vi "InitCA.vi"(11 "N-Back":u8) -> (3 "CA":T1(array[cluster]))   [LabVIEW 2020]
uses:
  Global Variables/Global N-Back Setting.vi
  Global Variables/Global Number of Indices.vi
panel:
  in  "New square":T2
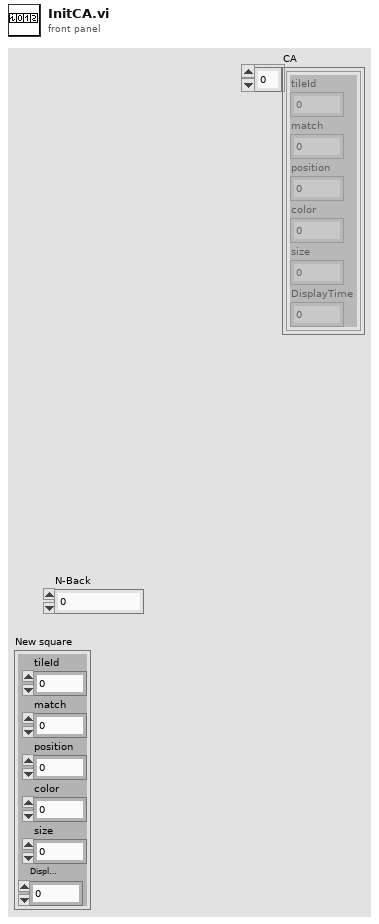
[diagram p1: front panel]
types:
  T1 = cluster{"tileId":i32, "match":i32, "position":i32, "color":u32, "size":i32, "DisplayTime":i32}[]
  T2 = cluster{"tileId":i32, "match":i32, "position":i32, "color":u32, "size":i32, "DisplayTime":i32}
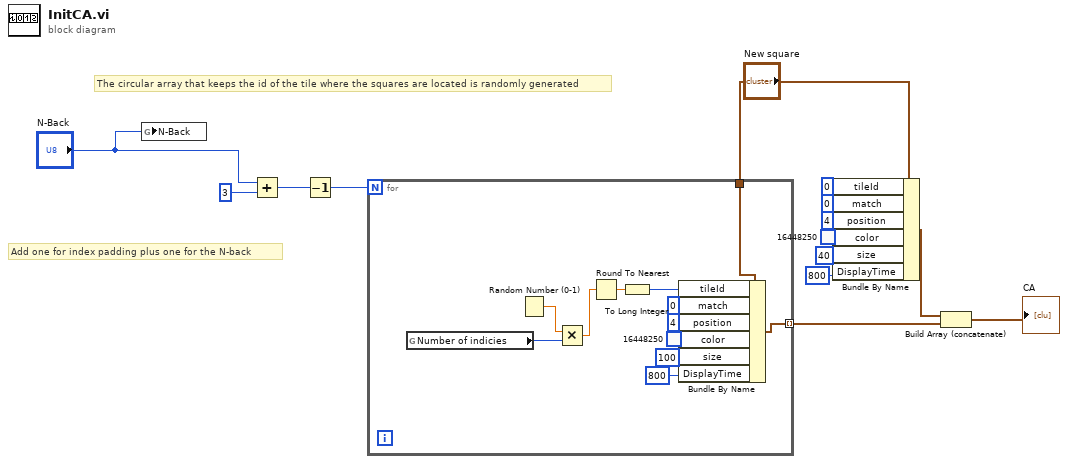
[diagram p0: block diagram]
diagram:
  # "The circular array that keeps the id of the tile where the squares are located is randomly generated"
  # "Add one for index padding plus one for the N-back"
  n1 = global write "Global N-Back Setting.vi" "N-Back"("N-Back") -> ()
  n2 = Add(x="N-Back", y=u8 3) -> (x+y=w12:u8)
  n3 = Decrement(x=w12) -> (x-1=w11:u8)
  n4 = for {
    N: w11 -> [_]
    tunnel: [w17] -> w5 mode=indexing
    tunnel: "New square" -> [w16]
    n5 = global read "Global Number of Indices.vi" "Number of indicies"() -> (w22:u8)
    n6 = Random Number (0-1)() -> (number: 0 to 1=w21:dbl)
    n7 = Multiply(x=w21, y=w22) -> (x*y=w20:dbl)
    n8 = Round To Nearest(number=w20) -> (nearest integer value=w19:dbl)
    n9 = To Long Integer(number=w19) -> (32bit integer=w18:i32)
    n10 = Bundle By Name(cluster=w16, "tileId"=w18, "match"=0, "position"=4, "color"=u32 16448250, "size"=100, "DisplayTime"=800) -> (w17:T2)
  }
  n11 = Bundle By Name(cluster="New square", "tileId"=0, "match"=0, "position"=4, "color"=u32 16448250, "size"=40, "DisplayTime"=800) -> (w6:T2)
  n12 = Build Array (concatenate)(w6, w5) -> (→"CA":T1)
